vi "niFpgaFFTPermutationSmallTemp.vi"(6 "perm switch":bool, 9 "stage switch":bool, 11 "bf data in":T1 {"x_r" format="%.16g"; "x_i" format="%.16g"; "y_r" format="%.16g"; "y_i" format="%.16g"}) -> (3 "bf data out":T1 {"x_r" format="%.16g"; "x_i" format="%.16g"; "y_r" format="%.16g"; "y_i" format="%.16g"})   [LabVIEW 2017]
uses:
  <vilib>/rvi/FXPMathLib/basic elements/FxpDiscreteDelay/XNode/nifxpmath_DiscreteDelay.xnode
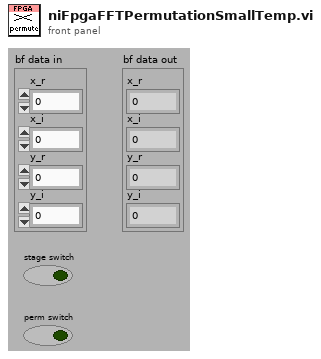
[diagram p1: front panel]
types:
  T1 = cluster{"x_r":fxp<+/-,16,1>, "x_i ":fxp<+/-,16,1>, "y_r ":fxp<+/-,16,1>, "y_i ":fxp<+/-,16,1>}
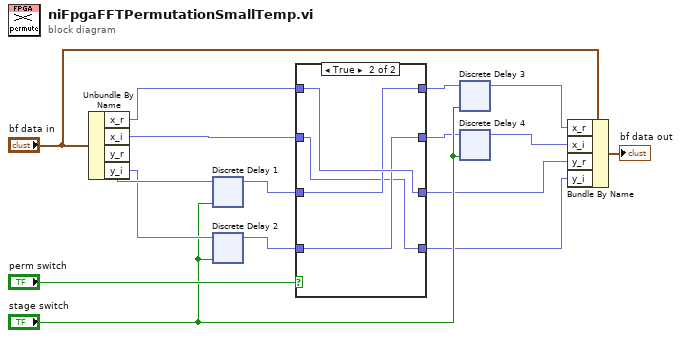
[diagram p0: block diagram]
diagram:
  n1 = Unbundle By Name("bf data in") -> ("x_r"=w14:fxp<+/-,16,1>, "x_i"=w13:fxp<+/-,16,1>, "y_r"=w12:fxp<+/-,16,1>, "y_i"=w11:fxp<+/-,16,1>)
  n2 = xnode "Discrete Delay 1"("D"=w12, "enable"="stage switch") -> ("Q"=w15:fxp<+/-,16,1>)
  n3 = xnode "Discrete Delay 2"("D"=w11, "enable"="stage switch") -> ("Q"=w9:fxp<+/-,16,1>)
  n4 = case shown="True" "perm switch" {
    tunnel: w15 -> [w20 w23]
    tunnel: [w18 w22] -> w6
    tunnel: [w20 w24] -> w3
    tunnel: w14 -> [w19 w24]
    tunnel: w13 -> [w18 w21]
    tunnel: [w19 w23] -> w7
    tunnel: w9 -> [w17 w22]
    tunnel: [w17 w21] -> w2
    frame False {
    }
    frame True {
    }
  }
  n5 = xnode "Discrete Delay 3"("D"=w7, "enable"="stage switch") -> ("Q"=w5:fxp<+/-,16,1>)
  n6 = xnode "Discrete Delay 4"("D"=w6, "enable"="stage switch") -> ("Q"=w4:fxp<+/-,16,1>)
  n7 = Bundle By Name(cluster="bf data in", "x_r"=w5, "x_i"=w4, "y_r"=w3, "y_i"=w2) -> (→"bf data out":T1)
